vi "SpeedAndBrakeValidate.vi"() -> ()   [LabVIEW 2016]
uses:
  <vilib>/Platform/TimedLoop/XDataNode/timing_clust.ctl
  <vilib>/Platform/TimedLoop/XDataNode/nitl_modes.ctl
  <vilib>/Platform/TimedLoop/XDataNode/wakeup.ctl
  <vilib>/FPGAPlugInAG/roboRIO/niLvFpga_Open_roboRIO.vi
  <vilib>/rvi/interface/common/dynamic/niFpgaDynamicAddResources.vi
  <vilib>/FPGAPlugInAG/Dynamic/niLvFpga_Reset_Dynamic.vi
  <vilib>/FPGAPlugInAG/Dynamic/niLvFpga_Run_Dynamic.vi
  <vilib>/Utility/error.llb/Error Cluster From Error Code.vi
  <vilib>/rvi/errors/niLvFpgaAdjustHostInterfaceError.vi
  <vilib>/FPGAPlugInAG/Dynamic/niLvFpga_Abort_Dynamic.vi
  <vilib>/FPGAPlugInAG/Dynamic/niLvFpga_Close_Dynamic.vi
  <vilib>/rvi/interface/nirviOpenFPGA/nirviOpenFPGA.xnode
  FPGA Bitfiles/AutoBikeProject_FPGATarget_AutoBikeFPGA_EwzLm8KNttI.lvbitx
  <vilib>/rvi/interface/nirviMethod/nirviMethod.xnode
  <vilib>/Platform/TimedLoop/XDataNode/XDataNode.xnode
  <vilib>/rvi/interface/nirviReadWriteControl/nirviReadWriteControl.xnode
  <vilib>/rvi/interface/nirviCloseFPGA/nirviCloseFPGA.xnode
  <vilib>/Platform/TimedLoop/XDataNode/XDNodeRunTimeDep.lvlib
  NiFpgaLv.dll
  <vilib>/rvi/interface/Simulation/niFpgaSimulationCallBeginRW.vi
panel:
  in  "Test choice":T1(ring)
  in  "Brake":bool
  out "Current velocity \nand reference":T2(graph)
  in  "Stop":bool
  out "Late loops":i32
  out "ERROR":sgl
  in  "Reference velocity in km/h":sgl=10.0
  out "Duty cycle (BW)":sgl
  out "Elapsed Time":i32 format="%<%H:%M:%S>t"
  out "error out":errorcluster
  # "SpeedTest1\nSpeed test without friction:\n0-30s -> 15km/h\n30-60s -> 8km/h\n60-90s ->12km/h\n90-120s ->15km/h"
  # "SpeedTest2\nSpeed test with constant friction, set to 1 on roller:\n0-30s -> 15km/h\n30-60s -> 8km/h\n60-90s ->12km/h\n90-120s ->15km/h"
  # "SpeedTest3\nSpeed test with varied friction, constant speed (12km/h):\n0-20s->0\n20-40s ->1\n40-60s ->2\n60-80s ->0\n80-100s->2\n100-120s->1"
  # "BrakeTest:\n0-15s -> 15km/h\nBRAKE!"
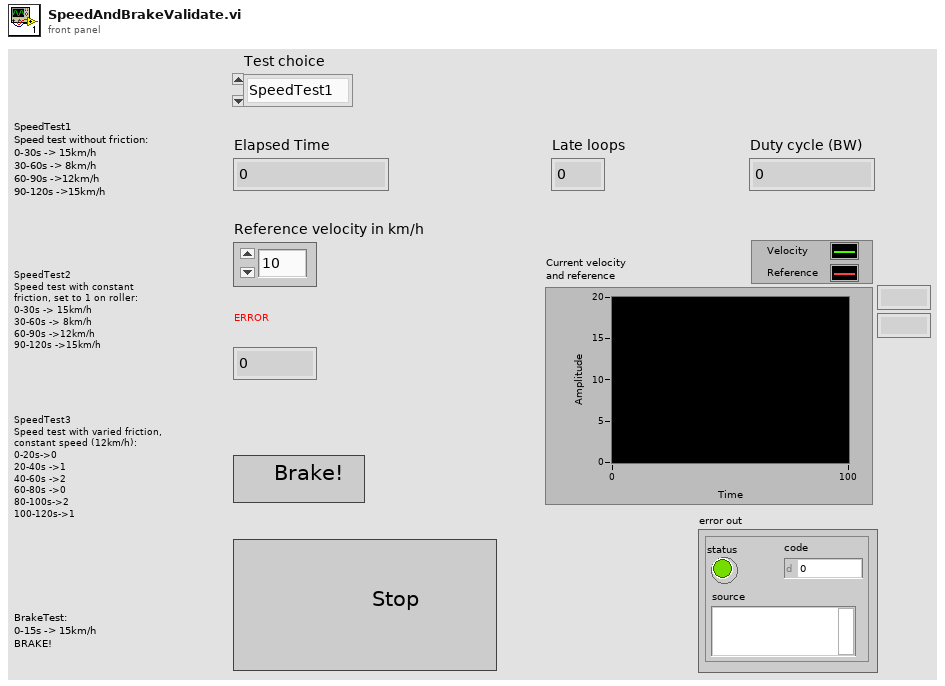
[diagram p1: front panel]
types:
  T1 = enum16{"SpeedTest1", "SpeedTest2", "SpeedTest3", "BrakeTest"}
  T2 = cluster{"Current velocity":sgl, "Reference velocity in km/h":sgl}
  T3 = enum16{"open", "open or create", "create or replace", "create", "open (read-only)"}
  T4 = typedef "XDNodeRunTimeDep.lvlib/timing_clust.ctl" = cluster{"Expected End [f-1]":u64, "Actual End [f-1]":u64, "Finished Late? [f-1]":bool, "Expected End [i-1]":u64, "Actual End [i-1]":u64, "Finished Late? [i-1]":bool, "Expected Start [i]":u64, "Actual Start [i]":u64, "Expected Start [f]":u64, "Actual Start [f]":u64, "Source Name":string, "Structure Name":string, "Period":i64, "Deadline":i64, "Offset":i64, "Start":i64, "Priority":i32, "Timeout":i32, "Mode":T5, "Wakeup Reason":T6, "Error":errorcluster, "Source Type":string, "Secondary Source Type":string, "Global End Time":u64, "Global Start Time":u64, "Frame Duration":u64, "Iteration Duration":u64, "Assigned CPU":i32, "I/O Scan Engine Mode":u32}
  T5 = typedef "XDNodeRunTimeDep.lvlib/nitl_modes.ctl" = enum32{"No Change", "Process missed periods, maintain original phase", "Discard missed periods, maintain original phase", "Process missed periods, ignore original phase", "Discard missed periods, ignore original phase"}
  T6 = typedef "XDNodeRunTimeDep.lvlib/wakeup.ctl" = enum32{"Normal", "Aborted", "Asynchronous wakeup", "Timing source error", "Timed loop error", "Timeout"}
  T7 = cluster{"Current speed":sgl, "Reference velocity in km/h":sgl}
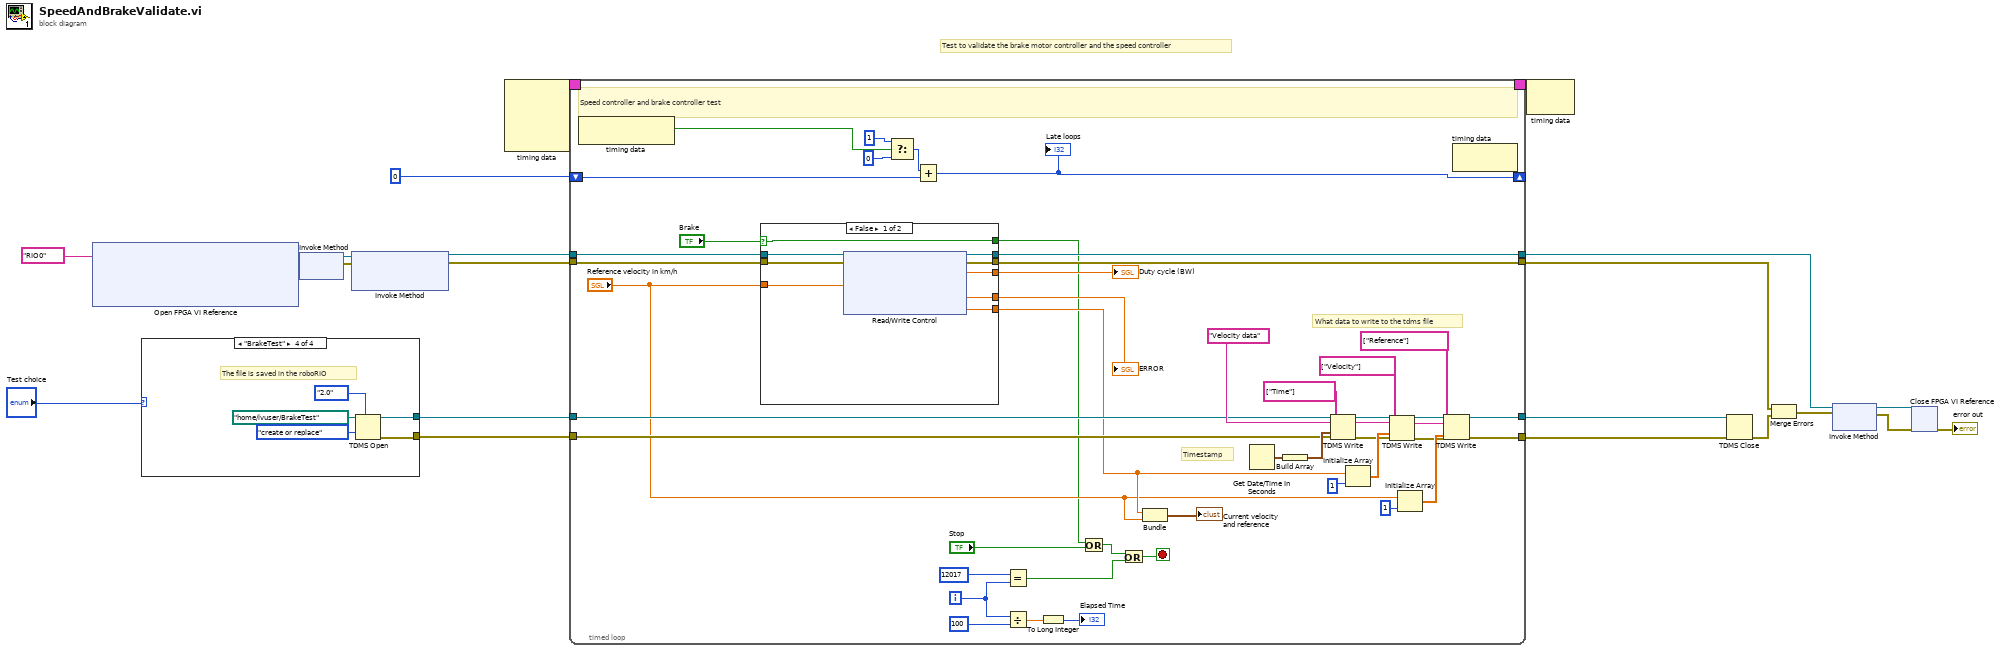
[diagram p0: block diagram]
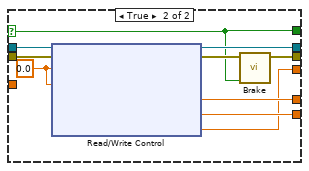
[diagram p2: hidden frame]
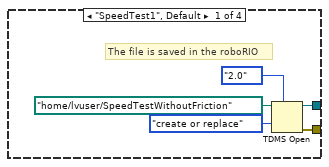
[diagram p3: hidden frame]
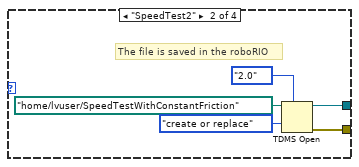
[diagram p4: hidden frame]
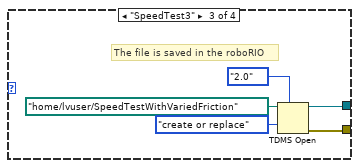
[diagram p5: hidden frame]
diagram:
  # "Test to validate the brake motor controller and the speed controller"
  n1 = xnode "Open FPGA VI Reference"("resource name"=tag "RIO0") -> ("FPGA VI Reference Out"=w22:refnum<k20>, "error out"=w10:errorcluster)  [unwired: 1 in]
  n2 = case shown="\"BrakeTest\"" "Test choice" {
    tunnel: [w24 w29 w34 w39] -> w11
    tunnel: [w23 w28 w33 w38] -> w8
    frame "SpeedTest1", Default {
      # "The file is saved in the roboRIO"
      n3 = TDMS Open(7:enum16{"1.0", "2.0"}."2.0" ("file format version (2.0)"), 10:T3."create or replace" ("operation (0:open)"), 11:path "/home/lvuser/SpeedTestWithoutFriction" ("file path")) -> (0:w23:errorcluster, 3:w24:refnum<k34>)  [unwired: 4 in]
    }
    frame "SpeedTest2" {
      # "The file is saved in the roboRIO"
      n4 = TDMS Open(7:enum16{"1.0", "2.0"}."2.0" ("file format version (2.0)"), 10:T3."create or replace" ("operation (0:open)"), 11:path "/home/lvuser/SpeedTestWithConstantFriction" ("file path")) -> (0:w28:errorcluster, 3:w29:refnum<k34>)  [unwired: 4 in]
    }
    frame "SpeedTest3" {
      # "The file is saved in the roboRIO"
      n5 = TDMS Open(7:enum16{"1.0", "2.0"}."2.0" ("file format version (2.0)"), 10:T3."create or replace" ("operation (0:open)"), 11:path "/home/lvuser/SpeedTestWithVariedFriction" ("file path")) -> (0:w33:errorcluster, 3:w34:refnum<k34>)  [unwired: 4 in]
    }
    frame "BrakeTest" {
      # "The file is saved in the roboRIO"
      n6 = TDMS Open(7:enum16{"1.0", "2.0"}."2.0" ("file format version (2.0)"), 10:T3."create or replace" ("operation (0:open)"), 11:path "/home/lvuser/BrakeTest" ("file path")) -> (0:w38:errorcluster, 3:w39:refnum<k34>)  [unwired: 4 in]
    }
  }
  n7 = xnode "Invoke Method"("FPGA VI Reference In"=w22, "error in"=w10) -> ("FPGA VI Reference Out"=w21:refnum<k20>, "error out"=w20:errorcluster)
  n8 = xnode "Invoke Method"("FPGA VI Reference In"=w21, "error in"=w20) -> ("FPGA VI Reference Out"=w13:refnum<k20>, "error out"=w7:errorcluster)  [unwired: 1 in]
  n9 = node-c288() -> (w2:T4)  [unwired: 4 in]
  n10 = timed-loop {
    timing: w2 -> [_]
    timing-out: [_] -> w1
    shift-right: [w79] -> _
    shift-left: 0 -> [w78]
    tunnel: [w66] -> w14
    tunnel: w13 -> [w62]
    tunnel: [w61] -> w12
    tunnel: w11 -> [w60]
    tunnel: [w57] -> w9
    tunnel: w8 -> [w56]
    tunnel: w7 -> [w55]
    tunnel: [w54] -> w6
    i -> [w49]
    stop <- w46 stop-if-true
    # "Timestamp"
    # "What data to write to the tdms file"
    # "Speed controller and brake controller test"
    n11 = node-c288() -> (w83:bool)  [unwired: 1 in]
    n12 = case shown="False" "Brake" {
      selector: "Brake" -> [w89 w100]
      tunnel: [w97 w104] -> w77
      tunnel: [w96 w98] -> w63
      tunnel: w62 -> [w95 w107]
      tunnel: [w94 w105] -> w61
      tunnel: w55 -> [w93 w106]
      tunnel: [w92 w101] -> w54
      tunnel: [w91 w103] -> w53
      tunnel: "Reference velocity in km/h" -> [w90 _]
      tunnel: [w89 w100] -> w44
      frame False {
        n13 = xnode "Read/Write Control"("FPGA VI Reference In"=w95, "error in"=w93, "Reference speed in km/h"=w90) -> ("FPGA VI Reference Out"=w94:refnum<k20>, "error out"=w92:errorcluster, "Duty cycle (BW)"=w96:sgl, "error"=w97:sgl, "Current speed"=w91:sgl)
      }
      frame True {
        w99 = sgl 0.0 ("Reference velocity in km/h")
        n14 = xnode "Read/Write Control"("FPGA VI Reference In"=w107, "error in"=w106, "Reference speed in km/h"=w99, "Duty cycle (BW)"=w99) -> ("FPGA VI Reference Out"=w105:refnum<k20>, "error out"=w102:errorcluster, "error"=w104:sgl, "Current speed"=w103:sgl, "Duty cycle (BW)"=w98:sgl)
        n15 = call "Brake.vi"("Brake!"=w100, "error in (no error)"=w102) -> ("error out"=w101:errorcluster)  [unwired: 9 in]
      }
    }
    "ERROR" <- w77
    "Duty cycle (BW)" <- w63
    n16 = Select(t=1, s=w83, f=0) -> (s? t:f=w80:i32)
    n17 = Add(x=w80, y=w78) -> (x+y=w79:i32)
    "Late loops" <- w79
    n18 = Equal?(x=12017, y=w49) -> (x = y?=w47:bool)
    n19 = Divide(x=w49, y=100) -> (x/y=w69:dbl)
    n20 = To Long Integer(number=w69) -> (32bit integer=→"Elapsed Time":i32)
    n21 = Or(x=w44, y="Stop") -> (x .or. y?=w48:bool)
    n22 = Or(x=w48, y=w47) -> (x .or. y?=w46:bool)
    n23 = Bundle("Current speed"=w53, "Reference velocity in km/h"="Reference velocity in km/h") -> (→"Current velocity \nand reference":T7)  [unwired: 1 in]
    n24 = Get Date/Time In Seconds() -> (seconds since 1Jan1904=w84:timestamp)
    n25 = Build Array(w84) -> (w85:timestamp[])
    n26 = TDMS Write(0:w60, 5:"Velocity data" ("group name in (Untitled)"), 7:string[] ["Time"] ("channel name(s) in (Untitled)"), 9:w85, 11:w56) -> (4:w59:refnum<k34>, 6:w65:string, 15:w64:errorcluster)  [unwired: 1 in, 1 out]
    n27 = Initialize Array(w53, 1 ("dimension size")) -> (w75:sgl[])
    n28 = TDMS Write(0:w59, 5:w65, 7:string[] ["Velocity"] ("channel name(s) in (Untitled)"), 9:w75, 11:w64) -> (4:w58:refnum<k34>, 6:w73:string, 15:w67:errorcluster)  [unwired: 1 in, 1 out]
    n29 = Initialize Array("Reference velocity in km/h", 1 ("dimension size")) -> (w71:sgl[])
    n30 = TDMS Write(0:w58, 5:w73, 7:string[] ["Reference"] ("channel name(s) in (Untitled)"), 9:w71, 11:w67) -> (4:w57:refnum<k34>, 15:w66:errorcluster)  [unwired: 1 in, 2 out]
    n31 = node-c288() -> ()  [unwired: 1 in, 1 out]
  }
  n32 = node-c288(w1) -> ()  [unwired: 1 out]
  n33 = TDMS Close(8:w14, 11:w9) -> (0:w5:errorcluster)  [unwired: 1 out]
  n34 = Merge Errors(w6, w5) -> (w4:errorcluster)
  n35 = xnode "Invoke Method"("FPGA VI Reference In"=w12, "error in"=w4) -> ("FPGA VI Reference Out"=w19:refnum<k20>, "error out"=w18:errorcluster)
  n36 = xnode "Close FPGA VI Reference"("FPGA VI Reference In"=w19, "error in"=w18) -> ("error out"=→"error out":errorcluster)
